vi "BallShear_Arduino-Continuous-Sampling-V3.vi"() -> ()   [LabVIEW 2013, in "LabVIEW Interface for Arduino.lvlib"]
doc: "This VI shows an example of using the continuous aquisition mode on the Arduino to aquire analog input data from a single input pin. The user can set the sample rate for the aquisition when the VI is first run. The maximum aquisition speed of the Arduino is 5KHZ. While this mode is turned on executing other LIFA commands will corrupt analog data. To use other LIFA commands turn continuous mode off first."
uses:
  <vilib>/LabVIEW Interface for Arduino/LabVIEW Interface for Arduino.lvlib
panel:
  out "output array":dbl[](array[numeric])
  in  "Array":dbl[](array[numeric])
  out "Waveform Chart":dbl[](graph)
  in  "Stop":bool
  in  "Sample Rate (HZ)":u16
  in  "Analog Input Pin":u8
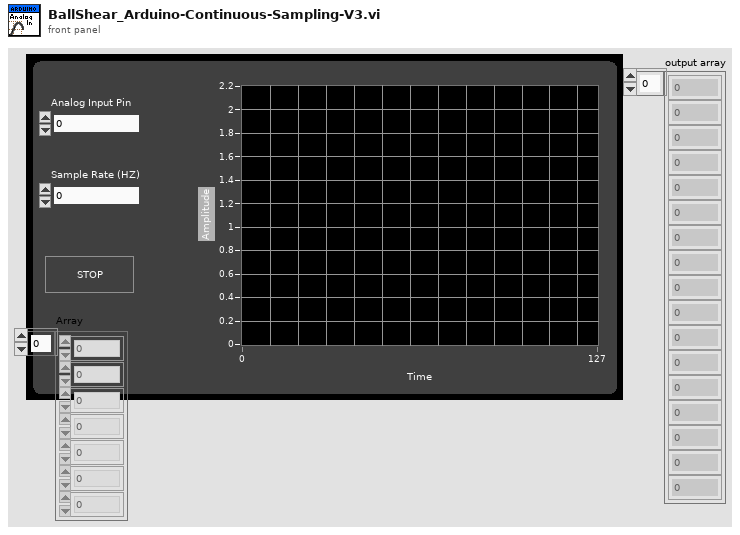
[diagram p1: front panel]
types:
  T1 = typedef "LabVIEW Interface for Arduino.lvlib/Arduino Resource.ctl" = cluster{"VISA resource":refnum<visa-resource-name>, "Board Type":T2, "Connection Type":enum8{"USB / Serial"}, "Bytes Per Packet (15)":u8}
  T2 = typedef "LabVIEW Interface for Arduino.lvlib/Board Type.ctl" = enum16{"Uno", "Dimuelanove w/Atmega 328", "Mega 2560"}
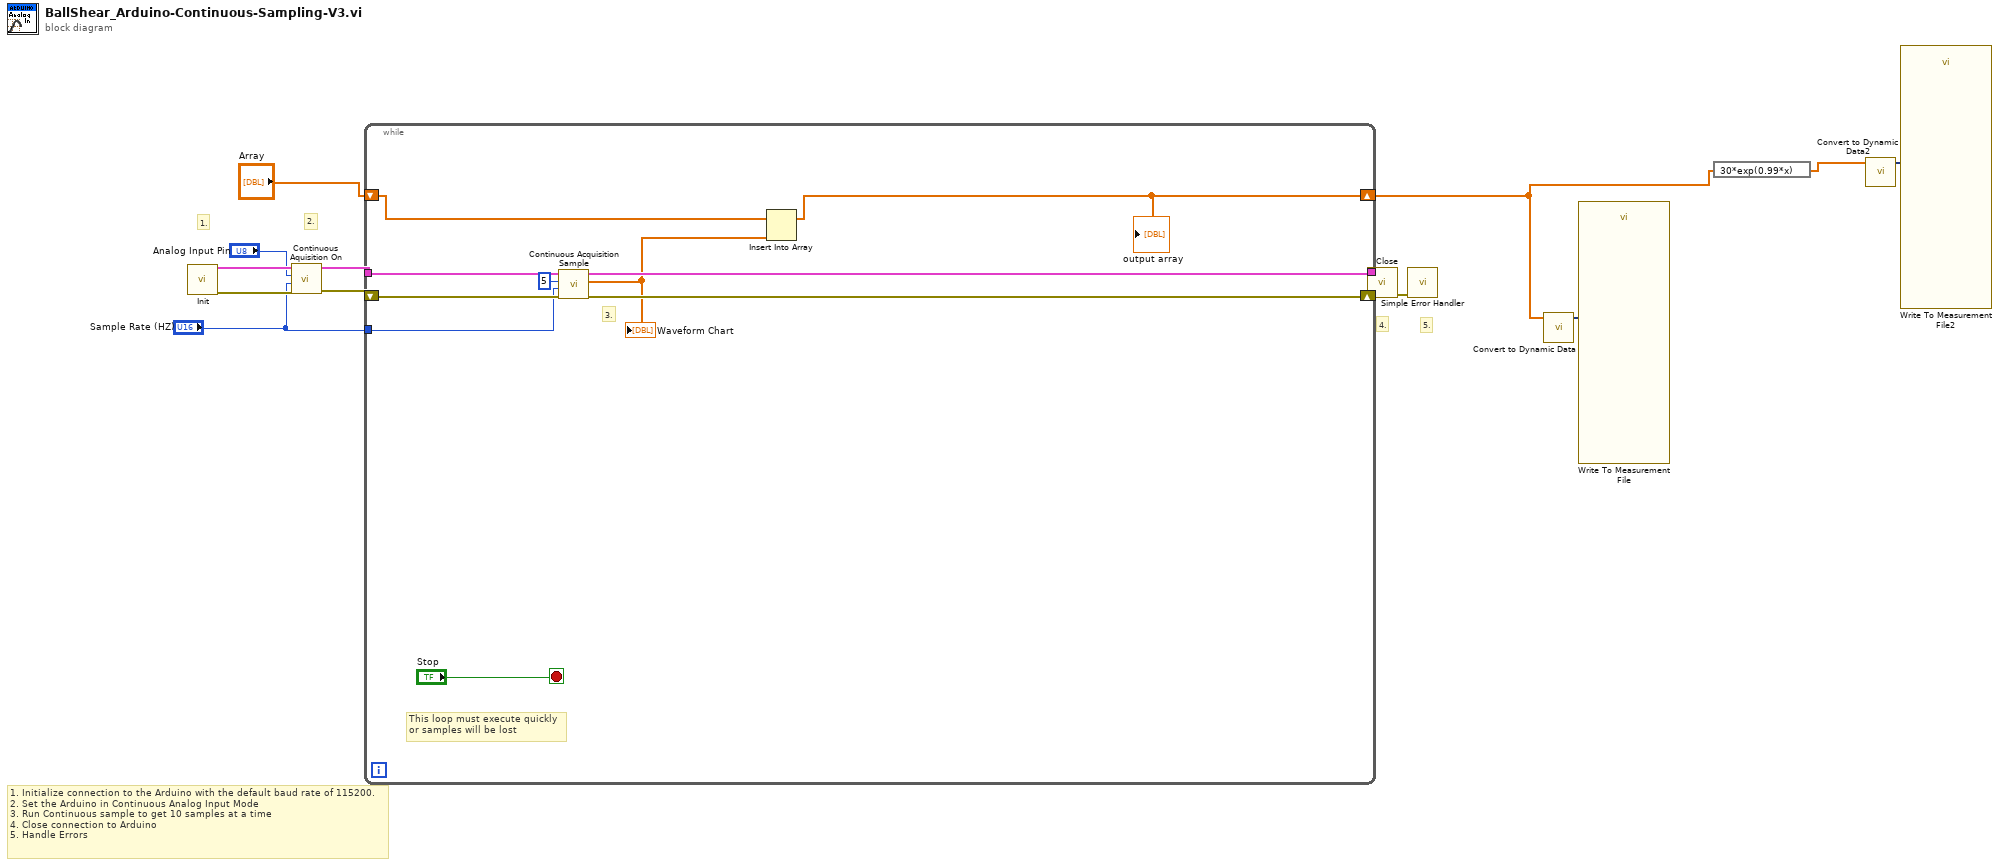
[diagram p0: block diagram]
diagram:
  # "5."
  # "4."
  # "2."
  # "1."
  # "1. Initialize connection to the Arduino with the default baud rate of 115200.\n2. Set the Arduino in Continuous Analog Input Mode\n3. Run Continuous sample to get 10 samples at a time\n4. Close connection to Arduino\n5. Handle Errors"
  n1 = call <vilib>:"Init.vi"() -> ("Arduino Resource"=w14:T1, "error out"=w7:errorcluster)  [unwired: 18 in]
  n2 = call <vilib>:"Continuous Aquisition On.vi"("error in"=w7, "Acquition Speed"="Sample Rate (HZ)", "Analog Input Pin"="Analog Input Pin", "Arduino Resource"=w14) -> ("error out"=w12:errorcluster, "Arduino Resource"=w13:T1)  [unwired: 6 in]
  n3 = while {
    tunnel: w13 -> [w23]
    tunnel: [w22] -> w11
    shift-right: [w21] -> w8
    shift-left: w12 -> [w20]
    tunnel: "Sample Rate (HZ)" -> [w18]
    shift-right: [w15] -> w3
    shift-left: "Array" -> [w17]
    stop <- "Stop" stop-if-true
    # "This loop must execute quickly\nor samples will be lost"
    # "3."
    n4 = call <vilib>:"Continuous Acquisition Sample.vi"("Arduino Resource"=w23, "Samples to Read"=u16 5, "Sample Rate (HZ)"=w18, "error in (no error)"=w20) -> ("Arduino Resource"=w22:T1, "Data"=w16:dbl[], "error out"=w21:errorcluster)  [unwired: 4 in]
    "Waveform Chart" <- w16
    n5 = Insert Into Array(array=w17, new element=w16) -> (w15:dbl[])  [unwired: 1 in]
    "output array" <- w15
  }
  n6 = call <vilib>:"Close.vi"("Arduino Resource"=w11, "error in"=w8) -> ("error out"=w10:errorcluster)  [unwired: 13 in]
  n7 = call <vilib>:"Simple Error Handler.vi"("error in (no error)"=w10) -> ()  [unwired: 4 in, 5 out]
  n8 = call "Convert to Dynamic Data"("Array"=w3) -> ("Dynamic Data Type"=w4:dynamicdata)  [unwired: 3 in]
  n9 = call "Write To Measurement File"("Signals"=w4) -> ()  [unwired: 16 in, 3 out]
  n10 = expression code="30*exp(0.99*x)"(w3) -> (w2:dbl[])
  n11 = call "Convert to Dynamic Data2"("Array"=w2) -> ("Dynamic Data Type"=w1:dynamicdata)  [unwired: 3 in]
  n12 = call "Write To Measurement File2"("Signals"=w1) -> ()  [unwired: 16 in, 3 out]
